vi "Host Main - 5172 Multi ch.vi"() -> ()   [LabVIEW 2021]
doc: "Use this VI as a template to design an application that acquires multiple records of data from the NI PXIe-5170R/5171R."
uses:
  <instrlib>/_niInstr/Multirecord Acquisition/Interface/v1/Host/Public/Requested Record Info.ctl
  <instrlib>/_niInstr/Multirecord Acquisition/Interface/v1/Host/Public/Full Record Status.ctl
  <instrlib>/_niInstr/Multirecord Acquisition/Interface/v1/Host/Public/Record State.ctl
  <instrlib>/_niInstr/Multirecord Acquisition/Interface/v1/Host/Public/Record Status.ctl
  <vilib>/FPGAPlugInAG/PXIe-5172 (8CH - 410T)/niLvFpga_Open_PXIe-5172 (8CH - 410T).vi
  <vilib>/rvi/interface/common/dynamic/niFpgaDynamicAddResources.vi
  <vilib>/FPGAPlugInAG/Dynamic/niLvFpga_Close_Dynamic.vi
  <vilib>/rvi/interface/nirviOpenFPGA/nirviOpenFPGA.xnode
  FPGA Bitfiles/5172 Multirecord Acquisition custom trigger.lvbitx
  <vilib>/rvi/interface/nirviCloseFPGA/nirviCloseFPGA.xnode
  Device Session/Device Session.lvclass
  <instrlib>/_niInstr/Multirecord Acquisition/Interface/v1/Host/niInstr Multirecord Acquisition v1 Host.lvclass
panel:
  out "Stop 2":bool
  out "Stop 1":bool
  out "Stop 0":bool
  in  "record number 3":u64
  out "record status 3":T1
  out "records done 3":u64
  out "current record status 3":T3
  out "requested records info 3":T4[](array[typedef])
  out "Waveform 2":T5(graph)
  out "overflow occurred 3":bool
  out "record status 2":T1
  out "records done 2":u64
  out "current record status 2":T3
  out "requested records info 2":T4[](array[typedef])
  out "Waveform 1":T5(graph)
  out "overflow occurred 2":bool
  in  "TrigCfg":T6(array[cluster])=[{"Center"=0.0, "Range"=0.2999999523162842}, {"Center"=0.0, "Range"=0.2999999523162842}, {"Center"=0.0, "Range"=0.2999999523162842}, {"Center"=0.0, "Range"=0.2999999523162842}, {"Center"=0.0, "Range"=0.2999999523162842}, {"Center"=0.0, "Range"=0.2999999523162842}, {"Center"=0.0, "Range"=0.2999999523162842}, {"Center"=0.0, "Range"=0.2999999523162842}]
  out "overflow occurred":bool
  in  "Stop":bool
  out "current record status":T3
  out "records done":u64
  out "record status":T1
  in  "pretrigger samples":u64=100
  out "Waveform 0":T5(graph)
  in  "number of samples":u64=5000
  in  "channels to configure":string="0,1,2"
  out "error out":errorcluster
  out "requested records info":T4[](array[typedef])
  in  "RIO Device":tag="PXI1Slot8"
  # "RIO Device"
  # "Channels"
  # "Acquisition Settings"
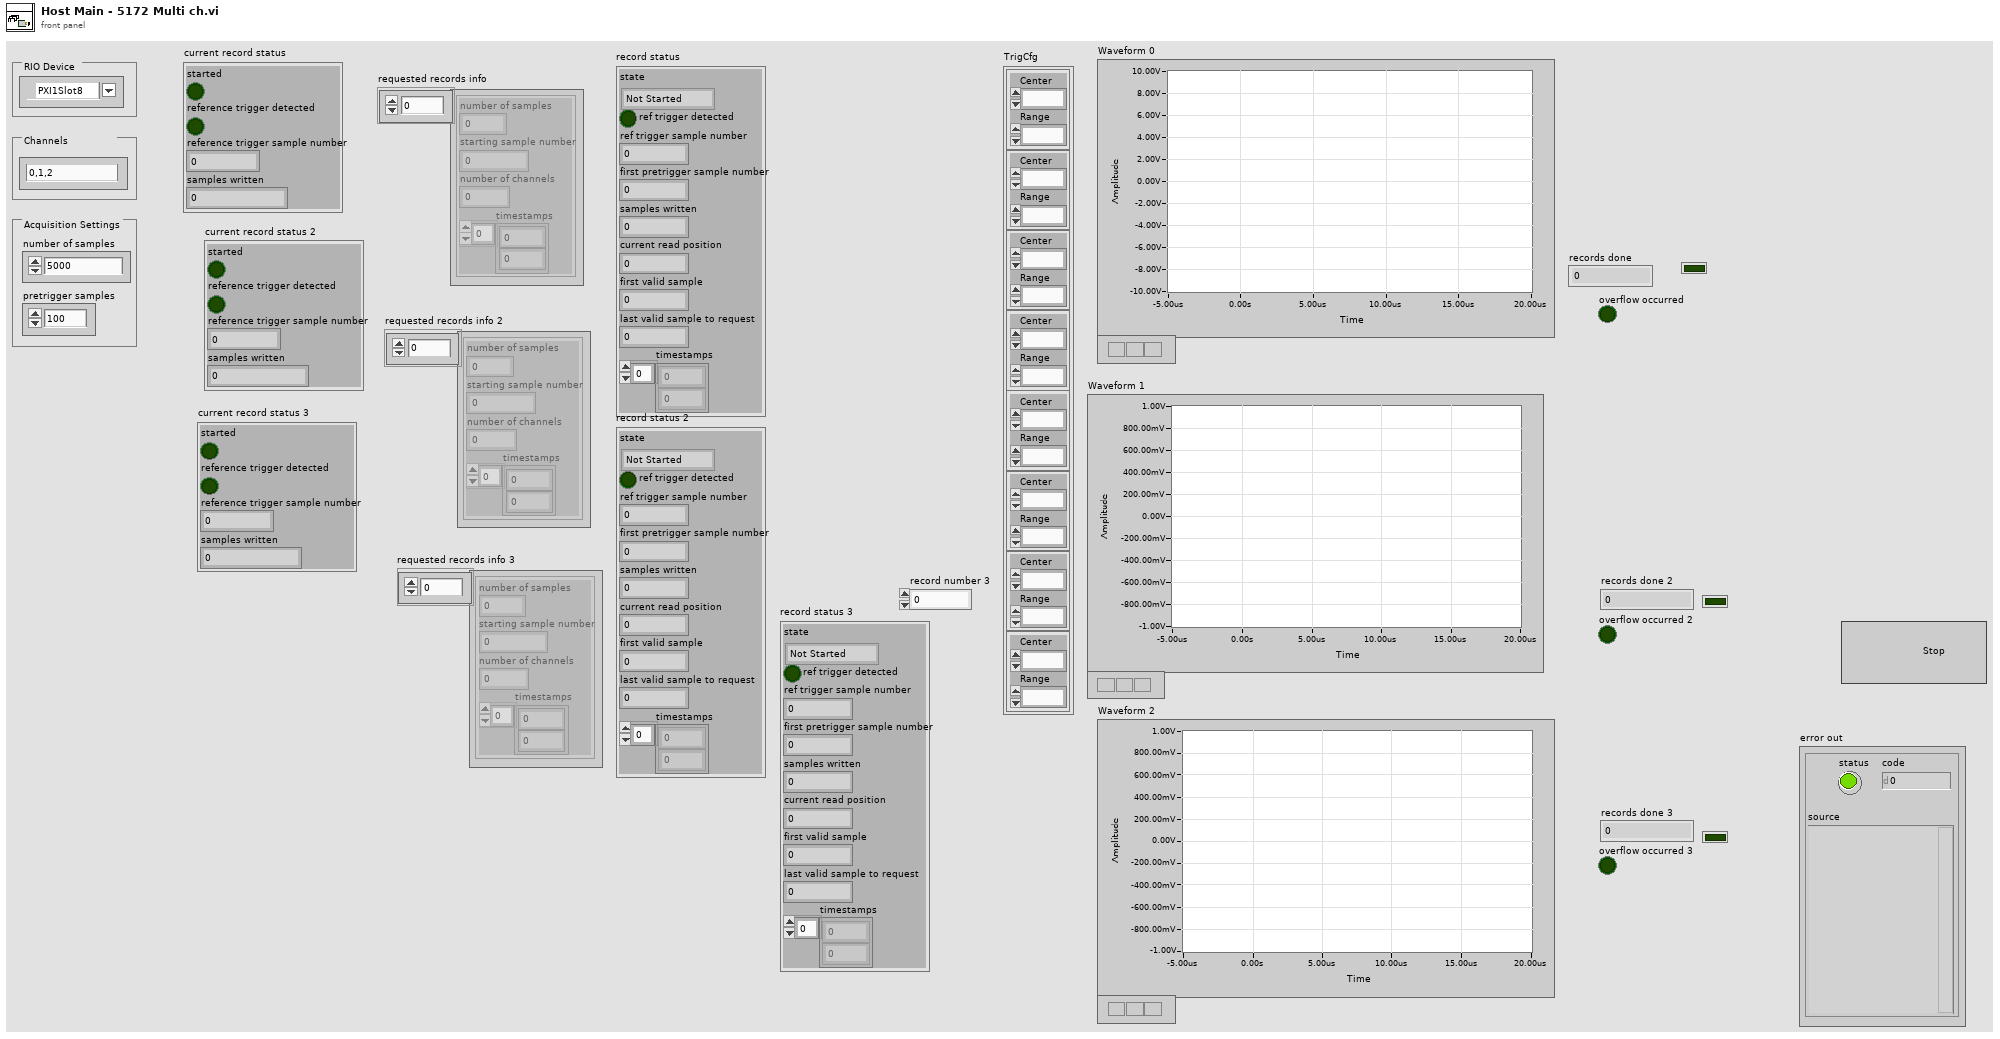
[diagram p1: front panel]
types:
  T1 = typedef "niInstr Multirecord Acquisition v1 Host.lvclass/Full Record Status.ctl" = cluster{"state":T2, "ref trigger detected":bool, "ref trigger sample number":u64, "first pretrigger sample number":u64, "samples written":u64, "current read position":u64, "first valid sample":u64, "last valid sample to request":u64, "timestamps":u64[]}
  T2 = typedef "niInstr Multirecord Acquisition v1 Host.lvclass/Record State.ctl" = enum16{"Not Started", "Being Acquired", "Completed", "Overwritten"}
  T3 = typedef "niInstr Multirecord Acquisition v1 Host.lvclass/Record Status.ctl" = cluster{"started":bool, "reference trigger detected":bool, "reference trigger sample number":u64, "samples written":u64}
  T4 = typedef "niInstr Multirecord Acquisition v1 Host.lvclass/Requested Record Info.ctl" = cluster{"number of samples":u64, "starting sample number":u64, "number of channels":u64, "timestamps":u64[]}
  T5 = cluster{"relativeX":dbl, "sample rate":dbl, "data in":dbl[]}[]
  T6 = cluster{"Center":fxp<+/-,24,1>, "Range":fxp<+,24,1>}[]
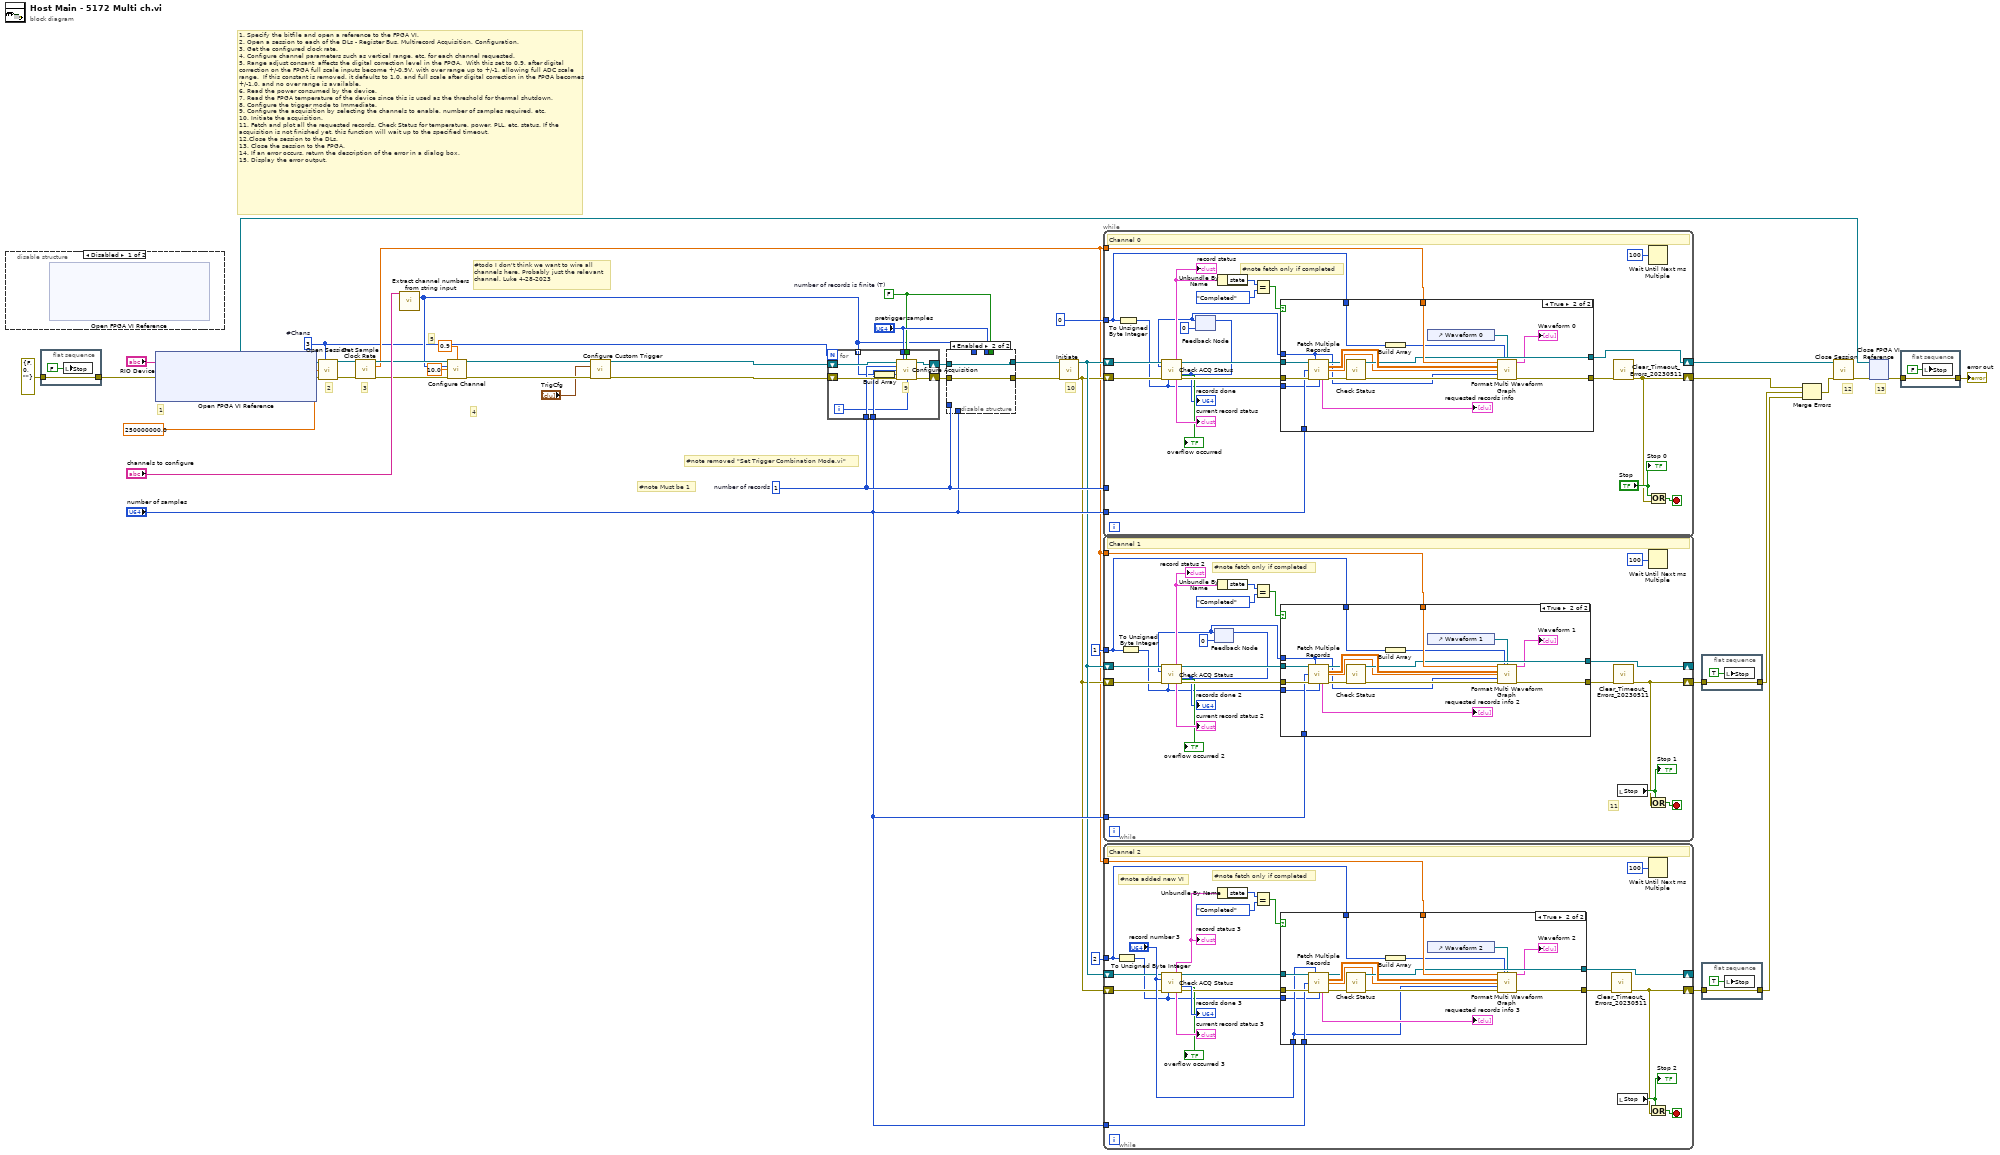
[diagram p0: block diagram]
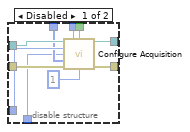
[diagram p2: hidden frame]
diagram:
  w2 = 3  # #Chans
  w34 = 250000000.0 items=["250 MHz"=250000000.0, "200 MHz"=200000000.0, "150 MHz"=150000000.0] ("onboard sample clock rate")
  w13 = u64 1  # number of records
  w14 = FALSE  # number of records is finite (T)
  # "#todo I don't think we want to wire all\nchannels here. Probably just the relevant\nchannel. Luke 4-28-2023"
  # "#note removed \"Set Trigger Combination Mode.vi\""
  # "#note Must be 1"
  # "5"
  # "13"
  # "12"
  # "11"
  # "10"
  # "4"
  # "3"
  # "1"
  # "2"
  # "1. Specify the bitfile and open a reference to the FPGA VI.\n2. Open a session to each of the DLs - Register Bus, Multirecord Acquisition, Configuration.\n3. Get the configured clock rate.\n4. Configure channel parameters such as vertical range, etc. for each channel requested.\n5. Range adjust consant  affects the digital correction level in the FPGA.  With this set to 0.9, after digital correction on the FPGA full scale inputs become +/-0.9V, with over range up to +/-1, allowing full ADC scale range.  If this constant is removed, it defaults to 1.0, and full scale after digital correction in the FPGA becomes +/-1.0, and no over range is available.\n6. Read the power consumed by the device.\n7. Read the FPGA temperature of the device since this is used as the threshold for thermal shutdown.\n8. Configure the trigger mode to Immediate.\n9. Configure the acquisition by selecting the channels to enable, number of samples required, etc.\n10. Initiate the acquisition.\n11. Fetch and plot all the requested records. Check Status for temperature, power, PLL, etc. status. If the acquisition is not finished yet, this function will wait up to the specified timeout.\n12.Close the session to the DLs.\n13. Close the session to the FPGA.\n14. If an error occurs, return the description of the error in a dialog box.\n15. Display the error output."
  n1 = disable-structure shown="Disabled" {
    frame Disabled {
      n2 = xnode "Open FPGA VI Reference"() -> ()  [unwired: 2 in, 2 out]
    }
    frame Enabled {
    }
  }
  n3 = flat-sequence {
    tunnel: errorcluster {"status"=FALSE, "code"=0, "source"=""} ("error out") -> [w45]
    tunnel: [w45] -> w21
    frame #0 {
      n4 = local write "Stop"(FALSE ("Stop")) -> ()
    }
  }
  n5 = xnode "Open FPGA VI Reference"("error in"=w21, "resource name"="RIO Device") -> ("FPGA VI Reference Out"=w37:refnum<k20>, "error out"=w29:errorcluster)
  n6 = call "Open Session.vi"("fpga reference in"=w37, "#Chans"=w2, "adc clock rate (Hz)"=w34, "error in"=w29) -> ("device session out"=w41:refnum<class "Device Session.lvclass">, "error out"=w42:errorcluster)  [unwired: 10 in]
  n7 = call "Get Sample Clock Rate.vi"("device session in"=w41, "error in"=w42) -> ("device session out"=w40:refnum<class "Device Session.lvclass">, "sample clock rate (Hz)"=w3:dbl, "error out"=w39:errorcluster)  [unwired: 11 in]
  n8 = call "Extract channel numbers from string input.vi"("channel input"="channels to configure") -> ("array of chans"=w12:u32[])  [unwired: 13 in, 1 out]
  n9 = call "Configure Channel.vi"("device session in"=w40, "range adjust"=0.9, "channels"=w12, "vertical range (Vpp)"=10.0, "error in"=w39) -> ("device session out"=w33:refnum<class "Device Session.lvclass">, "error out"=w32:errorcluster)  [unwired: 9 in]
  n10 = call "Configure Custom Trigger.vi"("device session in"=w33, "TrigCfg"="TrigCfg", "error in"=w32) -> ("device session out"=w31:refnum<class "Device Session.lvclass">, "error out"=w30:errorcluster)  [unwired: 11 in]
  n11 = for {
    N: w2 -> [_]
    tunnel: "pretrigger samples" -> [w53]
    tunnel: w14 -> [w52]
    tunnel: w13 -> [w51]
    tunnel: w12 -> [w50] mode=indexing
    tunnel: "number of samples" -> [w49]
    shift-right: [w55] -> w19
    shift-left: w31 -> [w57]
    shift-right: [w54] -> w17
    shift-left: w30 -> [w56]
    i -> [w48]
    # "9"
    n12 = Build Array(w50) -> (w47:u32[])
    n13 = call "Configure Acquisition.vi"("device session in"=w57, "pretrigger samples"=w53, "number of records is finite (T)"=w52, "number of records"=w51, "number of samples"=w49, "channels to store"=w47, "error in"=w56, "channel"=w48) -> ("device session out"=w55:refnum<class "Device Session.lvclass">, "error out"=w54:errorcluster)  [unwired: 5 in, 1 out]
  }
  n14 = disable-structure shown="Enabled" {
    disable-tunnel: w19 -> [w67 w69]
    disable-tunnel: [w66 w69] -> w18
    disable-tunnel: w17 -> [w65 w68]
    disable-tunnel: [w64 w68] -> w16
    disable-tunnel: "pretrigger samples" -> [w63 _]
    disable-tunnel: w14 -> [w62 _]
    disable-tunnel: w13 -> [w61 _]
    disable-tunnel: w12 -> [w60 _]
    disable-tunnel: "number of samples" -> [w58 _]
    frame Disabled {
      n15 = call "Configure Acquisition.vi"("device session in"=w67, "pretrigger samples"=w63, "number of records is finite (T)"=w62, "number of records"=w61, "number of samples"=w58, "channels to store"=w60, "error in"=w65, "channel"=u8 1) -> ("device session out"=w66:refnum<class "Device Session.lvclass">, "error out"=w64:errorcluster)  [unwired: 5 in, 1 out]
    }
    frame Enabled {
    }
  }
  n16 = call "Initiate.vi"("device session in"=w18, "error in"=w16) -> ("device session out"=w5:refnum<class "Device Session.lvclass">, "error out"=w4:errorcluster)  [unwired: 12 in]
  n17 = while {
    tunnel: "number of samples" -> [w79]
    tunnel: w3 -> [w78]
    shift-right: [w72] -> w27
    shift-left: w4 -> [w81]
    shift-right: [w74] -> w43
    shift-left: w5 -> [w82]
    tunnel: w13 -> [_]
    tunnel: u32 0 ("Numeric Control") -> [w75]
    stop <- w92 stop-if-true
    # "#note fetch only if completed"
    # "Channel 0"
    n18 = To Unsigned Byte Integer(number=w75) -> (unsigned 8bit integer=w70:u8)
    n19 = feedback #1(u64 0 ("record number")) -> (w71:u64)
    n20 = call "Check ACQ Status.vi"("device session in"=w82, "record number"=w71, "error in"=w81, "channel"=w70) -> ("record status"=w90:T1, "device session out"=w84:refnum<class "Device Session.lvclass">, "records done"=w77:u64, "overflow occurred"=→"overflow occurred":bool, "current record status"=→"current record status":T3, "error out"=w83:errorcluster)  [unwired: 6 in]
    "record status" <- w90
    "records done" <- w77
    n21 = feedback-in #1(w77) -> ()
    n22 = Unbundle By Name(w90) -> ("state"=w89:T2)
    n23 = Equal?(x=w89, y=Record_State."Completed" ("state")) -> (x = y?=w87:bool)
    n24 = case shown="True" w87 {
      tunnel: w78 -> [_ w111]
      tunnel: [w93 w109] -> w74
      tunnel: w75 -> [_ w96]
      tunnel: [w94 w104] -> w73
      tunnel: w84 -> [w93 w103]
      tunnel: w83 -> [w94 w102]
      tunnel: w79 -> [_ w101]
      tunnel: w71 -> [_ w100]
      tunnel: w70 -> [_ w97]
      frame False {
      }
      frame True {
        n25 = call "Fetch Multiple Records.vi"("device session in"=w103, "starting record"=w100, "number of samples"=w101, "error in"=w102, "channel"=w97) -> ("device session out"=w105:refnum<class "Device Session.lvclass">, "data"=w112:dbl[][], "relativeX (samples)"=w108:dbl[], "requested records info"=→"requested records info":T4[], "error out"=w107:errorcluster)  [unwired: 6 in]
        n26 = call "Check Status.vi"("device session in"=w105, "error in"=w107) -> ("device session out"=w109:refnum<class "Device Session.lvclass">, "error out"=w106:errorcluster)  [unwired: 12 in]
        n27 = Build Array(w96) -> (w95:u32[])
        n28 = control-ref of="Waveform 0"() -> (w99:refnum<vi>)
        n29 = call "Format Multi Waveform Graph.vi"("sample rate (Hz)"=w111, "array of chans"=w95, "waveform graph"=w99, "data in"=w112, "relativeX (samples)"=w108, "start record number"=w100, "error in"=w106) -> ("waveform out"=→"Waveform 0":T5, "error out"=w104:errorcluster)  [unwired: 7 in]
      }
    }
    n30 = call "Clear_Timeout_Errors_20230511.vi"("error in"=w73) -> ("error out"=w72:errorcluster)  [unwired: 10 in]
    n31 = Wait Until Next ms Multiple(millisecond multiple=u32 100) -> ()  [unwired: 1 out]
    n32 = Compound Arithmetic op=OR("Stop", w72) -> (w92:bool)
    "Stop 0" <- "Stop"
  }
  n33 = while {
    tunnel: "number of samples" -> [w122]
    tunnel: w3 -> [w121]
    shift-right: [w115] -> w25
    shift-left: w4 -> [w124]
    shift-right: [w135] -> _
    shift-left: w5 -> [w125]
    tunnel: u32 1 ("Numeric Control") -> [w119]
    stop <- w134 stop-if-true
    # "#note fetch only if completed"
    # "Channel 1"
    n34 = To Unsigned Byte Integer(number=w119) -> (unsigned 8bit integer=w113:u8)
    n35 = feedback #2(u64 0 ("record number")) -> (w114:u64)
    n36 = call "Check ACQ Status.vi"("device session in"=w125, "record number"=w114, "error in"=w124, "channel"=w113) -> ("record status"=w132:T1, "device session out"=w127:refnum<class "Device Session.lvclass">, "records done"=w118:u64, "overflow occurred"=→"overflow occurred 2":bool, "current record status"=→"current record status 2":T3, "error out"=w126:errorcluster)  [unwired: 6 in]
    "record status 2" <- w132
    "records done 2" <- w118
    n37 = feedback-in #2(w118) -> ()
    n38 = Unbundle By Name(w132) -> ("state"=w131:T2)
    n39 = Equal?(x=w131, y=Record_State."Completed" ("state")) -> (x = y?=w129:bool)
    n40 = case shown="True" w129 {
      tunnel: w121 -> [_ w154]
      tunnel: [w136 w152] -> w135
      tunnel: w119 -> [_ w138]
      tunnel: [w137 w147] -> w116
      tunnel: w127 -> [w136 w146]
      tunnel: w126 -> [w137 w145]
      tunnel: w122 -> [_ w144]
      tunnel: w114 -> [_ w143]
      tunnel: w113 -> [_ w140]
      frame False {
      }
      frame True {
        n41 = call "Fetch Multiple Records.vi"("device session in"=w146, "starting record"=w143, "number of samples"=w144, "error in"=w145, "channel"=w140) -> ("device session out"=w148:refnum<class "Device Session.lvclass">, "data"=w155:dbl[][], "relativeX (samples)"=w151:dbl[], "requested records info"=→"requested records info 2":T4[], "error out"=w150:errorcluster)  [unwired: 6 in]
        n42 = call "Check Status.vi"("device session in"=w148, "error in"=w150) -> ("device session out"=w152:refnum<class "Device Session.lvclass">, "error out"=w149:errorcluster)  [unwired: 12 in]
        n43 = Build Array(w138) -> (w139:u32[])
        n44 = control-ref of="Waveform 1"() -> (w142:refnum<vi>)
        n45 = call "Format Multi Waveform Graph.vi"("sample rate (Hz)"=w154, "array of chans"=w139, "waveform graph"=w142, "data in"=w155, "relativeX (samples)"=w151, "start record number"=w143, "error in"=w149) -> ("waveform out"=→"Waveform 1":T5, "error out"=w147:errorcluster)  [unwired: 7 in]
      }
    }
    n46 = call "Clear_Timeout_Errors_20230511.vi"("error in"=w116) -> ("error out"=w115:errorcluster)  [unwired: 10 in]
    n47 = local read "Stop"() -> (w117:bool)
    "Stop 1" <- w117
    n48 = Wait Until Next ms Multiple(millisecond multiple=u32 100) -> ()  [unwired: 1 out]
    n49 = Compound Arithmetic op=OR(w117, w115) -> (w134:bool)
  }
  n50 = while {
    tunnel: "number of samples" -> [w162]
    tunnel: w3 -> [w161]
    shift-right: [w157] -> w9
    shift-left: w4 -> [w164]
    shift-right: [w177] -> _
    shift-left: w5 -> [w165]
    tunnel: 2 ("Numeric Control") -> [w160]
    stop <- w176 stop-if-true
    # "#note fetch only if completed"
    # "#note added new VI"
    # "Channel 2"
    n51 = To Unsigned Byte Integer(number=w160) -> (unsigned 8bit integer=w156:u8)
    n52 = call "Check ACQ Status.vi"("device session in"=w165, "record number"="record number 3", "error in"=w164, "channel"=w156) -> ("record status"=w173:T1, "device session out"=w168:refnum<class "Device Session.lvclass">, "records done"=→"records done 3":u64, "overflow occurred"=→"overflow occurred 3":bool, "current record status"=→"current record status 3":T3, "error out"=w167:errorcluster)  [unwired: 6 in]
    "record status 3" <- w173
    n53 = Unbundle By Name(w173) -> ("state"=w172:T2)
    n54 = Equal?(x=w172, y=Record_State."Completed" ("state")) -> (x = y?=w170:bool)
    n55 = case shown="True" w170 {
      tunnel: w161 -> [_ w196]
      tunnel: [w178 w194] -> w177
      tunnel: w160 -> [_ w180]
      tunnel: [w179 w189] -> w158
      tunnel: w168 -> [w178 w188]
      tunnel: w167 -> [w179 w187]
      tunnel: w162 -> [_ w186]
      tunnel: "record number 3" -> [_ w185]
      tunnel: w156 -> [_ w182]
      frame False {
      }
      frame True {
        n56 = call "Fetch Multiple Records.vi"("device session in"=w188, "starting record"=w185, "number of samples"=w186, "error in"=w187, "channel"=w182) -> ("device session out"=w190:refnum<class "Device Session.lvclass">, "data"=w197:dbl[][], "relativeX (samples)"=w193:dbl[], "requested records info"=→"requested records info 3":T4[], "error out"=w192:errorcluster)  [unwired: 6 in]
        n57 = call "Check Status.vi"("device session in"=w190, "error in"=w192) -> ("device session out"=w194:refnum<class "Device Session.lvclass">, "error out"=w191:errorcluster)  [unwired: 12 in]
        n58 = Build Array(w180) -> (w181:i32[])
        n59 = control-ref of="Waveform 2"() -> (w184:refnum<vi>)
        n60 = call "Format Multi Waveform Graph.vi"("sample rate (Hz)"=w196, "array of chans"=w181, "waveform graph"=w184, "data in"=w197, "relativeX (samples)"=w193, "start record number"=w185, "error in"=w191) -> ("waveform out"=→"Waveform 2":T5, "error out"=w189:errorcluster)  [unwired: 7 in]
      }
    }
    n61 = call "Clear_Timeout_Errors_20230511.vi"("error in"=w158) -> ("error out"=w157:errorcluster)  [unwired: 10 in]
    n62 = local read "Stop"() -> (w159:bool)
    "Stop 2" <- w159
    n63 = Wait Until Next ms Multiple(millisecond multiple=u32 100) -> ()  [unwired: 1 out]
    n64 = Compound Arithmetic op=OR(w159, w157) -> (w176:bool)
  }
  n65 = flat-sequence {
    tunnel: w25 -> [w198]
    tunnel: [w198] -> w24
    frame #0 {
      n66 = local write "Stop"(TRUE ("Stop")) -> ()
    }
  }
  n67 = flat-sequence {
    tunnel: w9 -> [w200]
    tunnel: [w200] -> w8
    frame #0 {
      n68 = local write "Stop"(TRUE ("Stop")) -> ()
    }
  }
  n69 = Merge Errors(w27, w24, w8) -> (w26:errorcluster)
  n70 = call "Close Session.vi"("device session in"=w43, "error in"=w26) -> ("error out"=w36:errorcluster)  [unwired: 13 in]
  n71 = xnode "Close FPGA VI Reference"("FPGA VI Reference In"=w37, "error in"=w36) -> ("error out"=w23:errorcluster)
  n72 = flat-sequence {
    tunnel: w23 -> [w202]
    tunnel: [w202] -> w22
    frame #0 {
      n73 = local write "Stop"(FALSE ("Stop")) -> ()
    }
  }
  "error out" <- w22
